vi "SP - get item names (mclb).vi"(8 "error in (no error)":errorcluster, 11 "JSON string":string) -> (0 "error out":errorcluster, 3 "value":string)   [LabVIEW 2020, in "ui-testing.lvlib"]
doc: "copyright: Thomas Zilliox©"
uses:
  ui-testing.lvlib
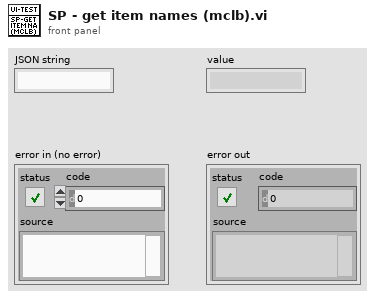
[diagram p1: front panel]
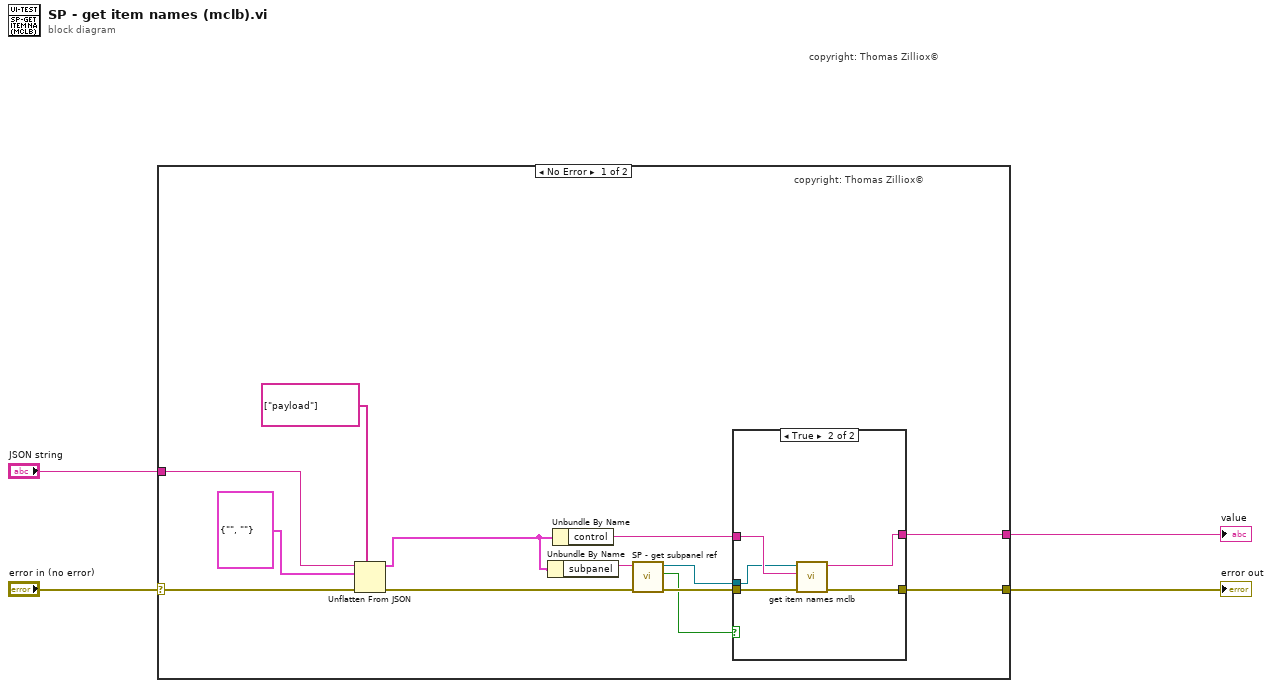
[diagram p0: block diagram]
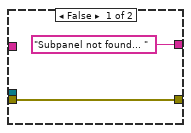
[diagram p2: hidden frame]
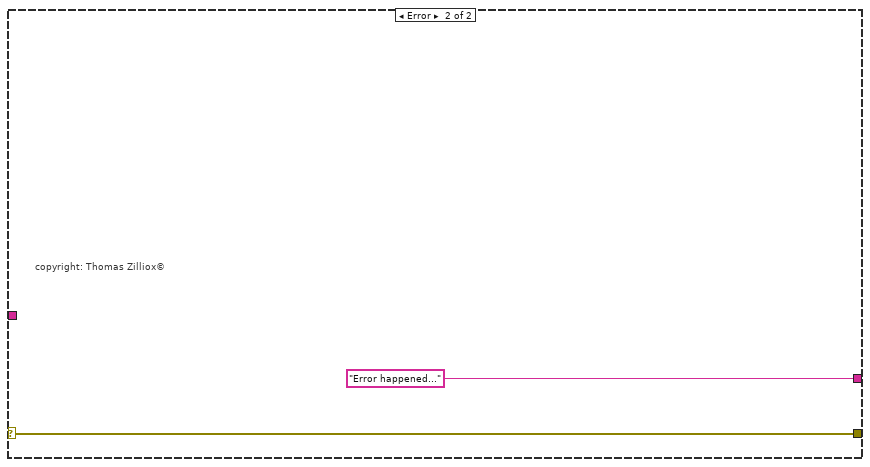
[diagram p3: hidden frame]
diagram:
  # "copyright: Thomas Zilliox©"
  n1 = case shown="No Error" "error in (no error)" {
    selector: "error in (no error)" -> [w15 w26]
    tunnel: "JSON string" -> [w14 _]
    tunnel: [w5 w26] -> w3
    tunnel: [w6 "Error happened..."] -> w2
    frame No Error {
      # "copyright: Thomas Zilliox©"
      n2 = Unflatten From JSON(path=string[] ["payload"], JSON string=w14, type and defaults=cluster{"subpanel":string, "control":string} {"subpanel"="", "control"=""}, error in (no error)=w15) -> (value=w7:cluster{"subpanel":string, "control":string}, error out=w8:errorcluster)  [unwired: 3 in]
      n3 = Unbundle By Name(w7) -> ("subpanel"=w13:string)
      n4 = Unbundle By Name(w7) -> ("control"=w9:string)
      n5 = call "SP - get subpanel ref.vi"("error in (no error)"=w8, "subpanel"=w13) -> ("error out"=w12:errorcluster, "subpanel found ?"=w10:bool, "subpanel VI ref"=w11:refnum<vi>)  [unwired: 6 in, 1 out]
      n6 = case shown="True" w10 {
        tunnel: [w19 w20] -> w5
        tunnel: w11 -> [_ w23]
        tunnel: w12 -> [w19 w21]
        tunnel: ["Subpanel not found... " ("result string") w22] -> w6
        tunnel: w9 -> [_ w24]
        frame False {
        }
        frame True {
          n7 = call "get item names mclb.vi"("error in (no error)"=w21, "Control label"=w24, "VI (Caller)"=w23) -> ("error out"=w20:errorcluster, "Item names"=w22:string)  [unwired: 7 in]
        }
      }
    }
    frame Error {
      # "copyright: Thomas Zilliox©"
    }
  }
  "error out" <- w3
  "value" <- w2
